vi "ex_4_4.vi"() -> ()   [LabVIEW 2020]
panel:
  in  "Sort by":enum16{"Row", "Column"}(ring)
  in  "Select Row":i32
  in  "Select Column":i32
  out "output array":dbl[][](array[numeric])
  in  "Array":dbl[][](array[numeric])
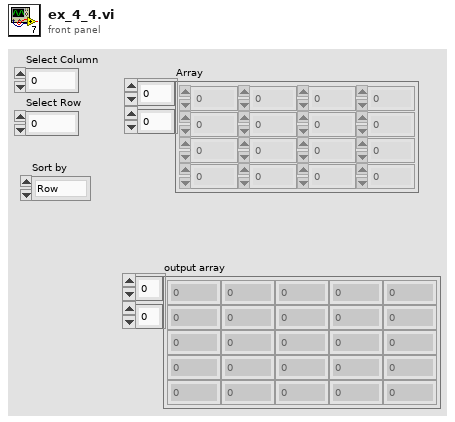
[diagram p1: front panel]
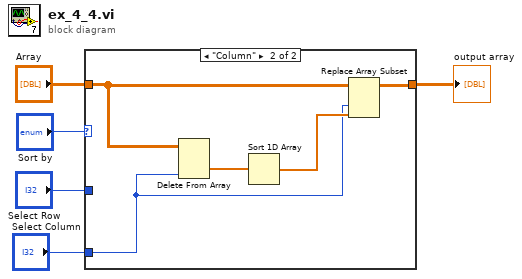
[diagram p0: block diagram]
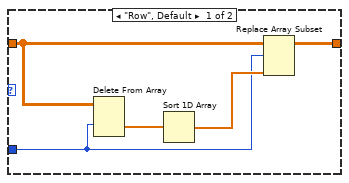
[diagram p2: hidden frame]
diagram:
  n1 = case shown="\"Column\"" "Sort by" {
    tunnel: [w8 w13] -> w4
    tunnel: "Array" -> [w7 w12]
    tunnel: "Select Row" -> [w6 _]
    tunnel: "Select Column" -> [_ w11]
    frame "Row", Default {
      n2 = Delete From Array(array=w7, index (row)=w6) -> (deleted portion=w9:dbl[])  [unwired: 2 in, 1 out]
      n3 = Sort 1D Array(array=w9) -> (sorted array=w10:dbl[])
      n4 = Replace Array Subset(array=w7, new element=w10, index (row)=w6) -> (w8:dbl[][])  [unwired: 1 in]
    }
    frame "Column" {
      n5 = Delete From Array(array=w12, index (col)=w11) -> (deleted portion=w14:dbl[])  [unwired: 2 in, 1 out]
      n6 = Sort 1D Array(array=w14) -> (sorted array=w15:dbl[])
      n7 = Replace Array Subset(array=w12, new element=w15, index (col)=w11) -> (w13:dbl[][])  [unwired: 1 in]
    }
  }
  "output array" <- w4
